vi "FlatToRichGreeter_MessageA.vi"(5 "OutputClusterType":T1, 11 "InputCluster":T2) -> (3 "OutputCluster":T1)   [LabVIEW 2019, in "Generated_server.lvlib"]
uses:
  Generated_server.lvlib
  Greeter_MessageA_Flat.ctl
  Greeter_MessageA.ctl
  Greeter_MessageA_oneof_a/Greeter_MessageA_oneof_a.lvclass
  Greeter_MessageA_oneof_a/Greeter_MessageA_oneof_a.lvclass/Greeter_MessageA_oneof_a.ctl
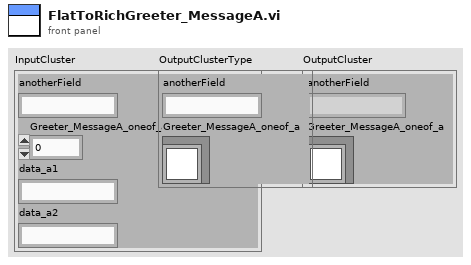
[diagram p1: front panel]
types:
  T1 = typedef "Generated_server.lvlib/Greeter_MessageA.ctl" = cluster{"anotherField":string, "Greeter_MessageA_oneof_a":refnum<class "Greeter_MessageA_oneof_a.lvclass">}
  T2 = typedef "Generated_server.lvlib/Greeter_MessageA_Flat.ctl" = cluster{"anotherField":string, "Greeter_MessageA_oneof_a_selected_index":i32, "data_a1":string, "data_a2":string}
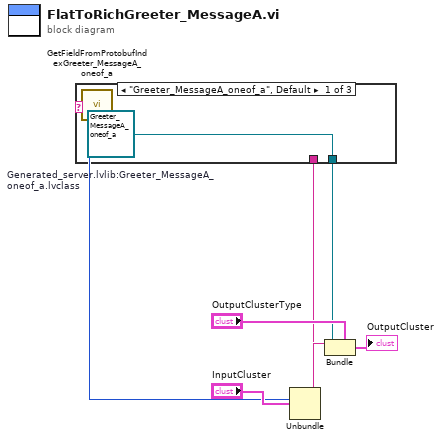
[diagram p0: block diagram]
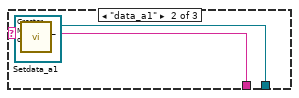
[diagram p2: hidden frame]
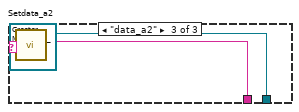
[diagram p3: hidden frame]
diagram:
  n1 = Unbundle "Unbundle"("InputCluster") -> ("anotherField"=w6:string, "Greeter_MessageA_oneof_a_selected_index"=w5:i32, "data_a1"=w2:string, "data_a2"=w1:string)
  n2 = call "GetFieldFromProtobufIndexGreeter_MessageA_oneof_a.vi"("protobuf index"=w5) -> ("oneof field name"=w4:string)
  n3 = case "Greeter_MessageA_oneof_a" shown="\"Greeter_MessageA_oneof_a\", Default" w4 {
    tunnel: [w10 w12 w15] -> w3
    tunnel: w2 -> [_ w13 _]
    tunnel: w1 -> [_ _ w16]
    frame "Greeter_MessageA_oneof_a", Default {
      w10 = refnum<class "Greeter_MessageA_oneof_a.lvclass"> refnum  # Generated_server.lvlib:Greeter_MessageA_oneof_a.lvclass
    }
    frame "data_a1" {
      n4 = call "Setdata_a1.vi"("Set_Val"=w13, "OneOfTemplate in"=refnum<class "Greeter_MessageA_oneof_a.lvclass"> refnum) -> ("OneOfTemplate out"=w12:refnum<class "Greeter_MessageA_oneof_a.lvclass">)  [unwired: 8 in, 1 out]
    }
    frame "data_a2" {
      n5 = call "Setdata_a2.vi"("Set_Val"=w16, "OneOfTemplate in"=refnum<class "Greeter_MessageA_oneof_a.lvclass"> refnum) -> ("OneOfTemplate out"=w15:refnum<class "Greeter_MessageA_oneof_a.lvclass">)  [unwired: 8 in, 1 out]
    }
  }
  n6 = Bundle "Bundle"(cluster="OutputClusterType", "anotherField"=w6, "Greeter_MessageA_oneof_a"=w3) -> (→"OutputCluster":T1)
